vi "Test Avoids Forbidden.vi"(11 "Test Case In":refnum<class "Numeric Keypad Forbidden Slot Test.lvclass">) -> (0 "error out":errorcluster, 3 "Test Case Out":refnum<class "Numeric Keypad Forbidden Slot Test.lvclass">)   [LabVIEW 2020, in "Numeric Keypad Forbidden Slot Test.lvclass"]
uses:
  Numeric Keypad Forbidden Slot Test.lvclass
  C:/Program Files (x86)/National Instruments/LabVIEW 2020/vi.lib/Astemes/LUnit/Test Case.lvclass
  Numeric Keypad Forbidden Slot Test.lvclass/Numeric Keypad Forbidden Slot Test.ctl
  <vilib>/Astemes/LUnit/Test Case.lvclass/Test Case.ctl
  92924050-e759-45e2-b7a4-5e1b8a8c74f9.vi
  <vilib>/Astemes/LUnit/Palette/Fail If.vi
  <vilib>/Astemes/LUnit/Append Pass Result.vi
  <vilib>/Astemes/LUnit/Append Fail Result.vi
  <vilib>/Astemes/LUnit/Run In UI.vi
  <vilib>/Utility/error.llb/Clear Errors.vi
  Numeric Keypad/Numeric Keypad.lvclass
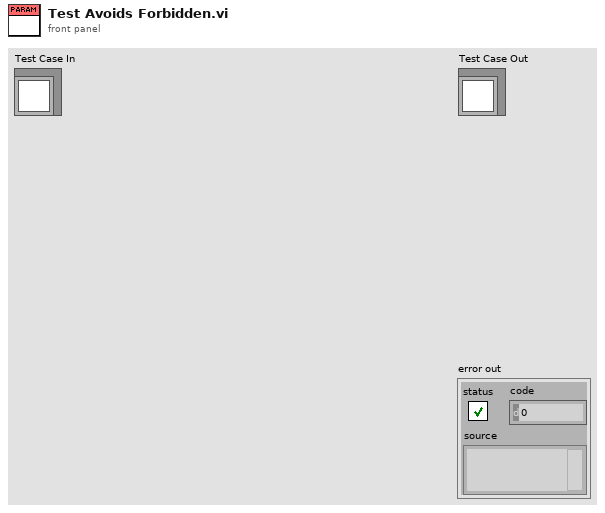
[diagram p1: front panel]
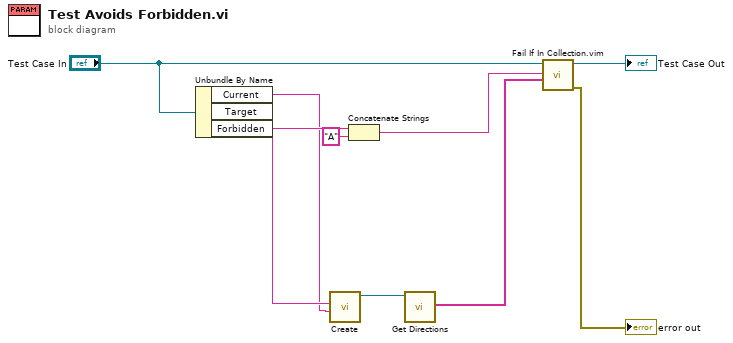
[diagram p0: block diagram]
diagram:
  n1 = Unbundle By Name("Test Case In") -> ("Current"=w3:string, "Target"=w4:string, "Forbidden"=w6:string)
  n2 = call "Create.vi"("Current"=w3, "Input"=w4) -> ("Proto"=w7:refnum<class "Numeric Keypad.lvclass">)  [unwired: 9 in]
  n3 = Concatenate Strings(w6, "A" ("string")) -> (w2:string)
  n4 = call "Get Directions.vi"("Proto in"=w7) -> ("Directional Button Presses"=w5:string[])  [unwired: 9 in, 1 out]
  n5 = call "Fail If In Collection.vim"("Collection"=w5, "Element"=w2, "LUnit Test Case In"="Test Case In") -> ("error out"=→"error out":errorcluster, "LUnit Test Case Out"=→"Test Case Out":refnum<class "Numeric Keypad Forbidden Slot Test.lvclass">)  [unwired: 7 in]
